vi "WILT Agilent Data To Main Display.vi"(0 "GUI Aisle 4":T3[](array[typedef]) {"Night Cycle Count" format="%04d"; "Day Cycle Count" format="%04d"}, 5 "GUI Aisle 3":T3[](array[typedef]) {"Night Cycle Count" format="%04d"; "Day Cycle Count" format="%04d"}, 7 "GUI Aisle 2":T3[](array[typedef]) {"Night Cycle Count" format="%04d"; "Day Cycle Count" format="%04d"}, 9 "GUI Aisle 1 (SLAT)":T3[](array[typedef]) {"Night Cycle Count" format="%04d"; "Day Cycle Count" format="%04d"}, 11 "Error In":errorcluster, 12 "GUI Aisle 1A (SLAT)":T3[](array[typedef]) {"Night Cycle Count" format="%04d"; "Day Cycle Count" format="%04d"}, 13 "Data Array":T1) -> (3 "Agilent Failure":bool, 4 "GUI Aisle 4 Out":T3[](array[typedef]) {"Night Cycle Count" format="%04d"; "Day Cycle Count" format="%04d"}, 6 "GUI Aisle 3 Out":T3[](array[typedef]) {"Night Cycle Count" format="%04d"; "Day Cycle Count" format="%04d"}, 8 "GUI Aisle 2 Out":T3[](array[typedef]) {"Night Cycle Count" format="%04d"; "Day Cycle Count" format="%04d"}, 10 "GUI Aisle 1 (SLAT) Out":T3[](array[typedef]) {"Night Cycle Count" format="%04d"; "Day Cycle Count" format="%04d"}, 14 "GUI Aisle 1A (SLAT) Out":T3[](array[typedef]) {"Night Cycle Count" format="%04d"; "Day Cycle Count" format="%04d"}, 15 "Error Out":errorcluster)   [LabVIEW 2016]
uses:
  Type Definitions/WILT Dryer.ctl
  Type Definitions/WILT Dryer Details.ctl
  Type Definitions/WILT Agilent Channel Definition.ctl
  Type Definitions/WILT DAQ Data.ctl
  Type Definitions/WILT Agilent Data Cluster.ctl
  Type Definitions/WILT Aisle Number.ctl
panel:
  in  "Test Data Only!!":T2[](array[typedef])=[{"Channel"="101", "Station"="1", "Label"="L1 Current", "Agilent Station"="1", "Data"=0.0}, {"Channel"="102", "Station"="1", "Label"="L2 Current", "Agilent Station"="1", "Data"=0.0}, {"Channel"="103", "Station"="2", "Label"="L1 Current", "Agilent Station"="1", "Data"=0.0}, {"Channel"="104", "Station"="2", "Label"="L2 Current", "Agilent Station"="1", "Data"=0.0}, {"Channel"="105", "Station"="3", "Label"="L1 Current", "Agilent Station"="1", "Data"=0.0}, {"Channel"="106", "Station"="3", "Label"="L2 Current", "Agilent Station"="1", "Data"=0.0}, {"Channel"="107", "Station"="4", "Label"="L1 Current", "Agilent Station"="1", "Data"=0.0}, {"Channel"="108", "Station"="4", "Label"="L2 Current", "Agilent Station"="1", "Data"=0.0}, {"Channel"="109", "Station"="5", "Label"="L1 Current", "Agilent Station"="1", "Data"=0.0}, {"Channel"="110", "Station"="5", "Label"="L2 Current", "Agilent Station"="1", "Data"=0.0}, {"Channel"="111", "Station"="6", "Label"="L1 Current", "Agilent Station"="1", "Data"=0.0}, {"Channel"="112", "Station"="6", "Label"="L2 Current", "Agilent Station"="1", "Data"=0.0}, {"Channel"="113", "Station"="7", "Label"="L1 Current", "Agilent Station"="1", "Data"=0.0}, {"Channel"="114", "Station"="7", "Label"="L2 Current", "Agilent Station"="1", "Data"=0.0}, {"Channel"="115", "Station"="8", "Label"="L1 Current", "Agilent Station"="1", "Data"=0.0}, {"Channel"="116", "Station"="8", "Label"="L2 Current", "Agilent Station"="1", "Data"=0.0}, {"Channel"="201", "Station"="9", "Label"="L1 Current", "Agilent Station"="1", "Data"=0.0}, {"Channel"="202", "Station"="9", "Label"="L2 Current", "Agilent Station"="1", "Data"=0.0}, {"Channel"="203", "Station"="10", "Label"="L1 Current", "Agilent Station"="1", "Data"=0.0}, {"Channel"="204", "Station"="10", "Label"="L2 Current", "Agilent Station"="1", "Data"=0.0}, {"Channel"="205", "Station"="11", "Label"="L1 Current", "Agilent Station"="1", "Data"=0.0}, {"Channel"="206", "Station"="11", "Label"="L2 Current", "Agilent Station"="1", "Data"=0.0}, {"Channel"="207", "Station"="12", "Label"="L1 Current", "Agilent Station"="1", "Data"=0.0}, {"Channel"="208", "Station"="12", "Label"="L2 Current", "Agilent Station"="1", "Data"=0.0}, {"Channel"="209", "Station"="13", "Label"="L1 Current", "Agilent Station"="1", "Data"=0.0}, {"Channel"="210", "Station"="13", "Label"="L2 Current", "Agilent Station"="1", "Data"=0.0}, {"Channel"="211", "Station"="14", "Label"="L1 Current", "Agilent Station"="1", "Data"=0.0}, {"Channel"="212", "Station"="14", "Label"="L2 Current", "Agilent Station"="1", "Data"=0.0}, {"Channel"="213", "Station"="15", "Label"="L1 Current", "Agilent Station"="1", "Data"=0.0}, {"Channel"="214", "Station"="15", "Label"="L2 Current", "Agilent Station"="1", "Data"=0.0}, {"Channel"="215", "Station"="16", "Label"="L1 Current", "Agilent Station"="1", "Data"=0.0}, {"Channel"="216", "Station"="16", "Label"="L2 Current", "Agilent Station"="1", "Data"=0.0}, {"Channel"="301", "Station"="17", "Label"="L1 Current", "Agilent Station"="1", "Data"=0.0}, {"Channel"="302", "Station"="17", "Label"="L2 Current", "Agilent Station"="1", "Data"=0.0}, {"Channel"="303", "Station"="18", "Label"="L1 Current", "Agilent Station"="1", "Data"=0.0}, {"Channel"="304", "Station"="18", "Label"="L2 Current", "Agilent Station"="1", "Data"=0.0}, {"Channel"="305", "Station"="19", "Label"="L1 Current", "Agilent Station"="1", "Data"=0.0}, {"Channel"="306", "Station"="19", "Label"="L2 Current", "Agilent Station"="1", "Data"=0.0}, {"Channel"="307", "Station"="20", "Label"="L1 Current", "Agilent Station"="1", "Data"=0.0}, {"Channel"="308", "Station"="20", "Label"="L2 Current", "Agilent Station"="1", "Data"=0.0}, {"Channel"="309", "Station"="21", "Label"="L1 Current", "Agilent Station"="1", "Data"=0.0}, {"Channel"="310", "Station"="21", "Label"="L2 Current", "Agilent Station"="1", "Data"=0.0}, {"Channel"="311", "Station"="22", "Label"="L1 Current", "Agilent Station"="1", "Data"=0.0}, {"Channel"="312", "Station"="22", "Label"="L2 Current", "Agilent Station"="1", "Data"=0.0}, {"Channel"="313", "Station"="23", "Label"="L1 Current", "Agilent Station"="1", "Data"=0.0}, {"Channel"="314", "Station"="23", "Label"="L2 Current", "Agilent Station"="1", "Data"=0.0}, {"Channel"="315", "Station"="24", "Label"="L1 Current", "Agilent Station"="1", "Data"=0.0}, {"Channel"="316", "Station"="24", "Label"="L2 Current", "Agilent Station"="1", "Data"=0.0}, {"Channel"="101", "Station"="25", "Label"="L1 Current", "Agilent Station"="2", "Data"=0.0}, {"Channel"="102", "Station"="25", "Label"="L2 Current", "Agilent Station"="2", "Data"=0.0}, {"Channel"="103", "Station"="26", "Label"="L1 Current", "Agilent Station"="2", "Data"=0.0}, {"Channel"="104", "Station"="26", "Label"="L2 Current", "Agilent Station"="2", "Data"=0.0}, {"Channel"="105", "Station"="27", "Label"="L1 Current", "Agilent Station"="2", "Data"=0.0}, {"Channel"="106", "Station"="27", "Label"="L2 Current", "Agilent Station"="2", "Data"=0.0}, {"Channel"="107", "Station"="28", "Label"="L1 Current", "Agilent Station"="2", "Data"=0.0}, {"Channel"="108", "Station"="28", "Label"="L2 Current", "Agilent Station"="2", "Data"=0.0}, {"Channel"="109", "Station"="29", "Label"="L1 Current", "Agilent Station"="2", "Data"=0.0}, {"Channel"="110", "Station"="29", "Label"="L2 Current", "Agilent Station"="2", "Data"=0.0}, {"Channel"="111", "Station"="30", "Label"="L1 Current", "Agilent Station"="2", "Data"=0.0}, {"Channel"="112", "Station"="30", "Label"="L2 Current", "Agilent Station"="2", "Data"=0.0}, {"Channel"="113", "Station"="31", "Label"="L1 Current", "Agilent Station"="2", "Data"=0.0}, {"Channel"="114", "Station"="31", "Label"="L2 Current", "Agilent Station"="2", "Data"=0.0}, {"Channel"="115", "Station"="32", "Label"="L1 Current", "Agilent Station"="2", "Data"=0.0}, {"Channel"="116", "Station"="32", "Label"="L2 Current", "Agilent Station"="2", "Data"=0.0}, {"Channel"="201", "Station"="5", "Label"="Volts", "Agilent Station"="2", "Data"=0.0}, {"Channel"="202", "Station"="6", "Label"="Volts", "Agilent Station"="2", "Data"=0.0}, {"Channel"="203", "Station"="7", "Label"="Volts", "Agilent Station"="2", "Data"=0.0}, {"Channel"="204", "Station"="8", "Label"="Volts", "Agilent Station"="2", "Data"=0.0}, {"Channel"="205", "Station"="9", "Label"="Volts", "Agilent Station"="2", "Data"=0.0}, {"Channel"="206", "Station"="10", "Label"="Volts", "Agilent Station"="2", "Data"=0.0}, {"Channel"="207", "Station"="11", "Label"="Volts", "Agilent Station"="2", "Data"=0.0}, {"Channel"="208", "Station"="12", "Label"="Volts", "Agilent Station"="2", "Data"=0.0}, {"Channel"="209", "Station"="13", "Label"="Volts", "Agilent Station"="2", "Data"=0.0}, {"Channel"="210", "Station"="14", "Label"="Volts", "Agilent Station"="2", "Data"=0.0}, {"Channel"="211", "Station"="21-23", "Label"="Volts", "Agilent Station"="2", "Data"=0.0}, {"Channel"="212", "Station"="24-26", "Label"="Volts", "Agilent Station"="2", "Data"=0.0}, {"Channel"="213", "Station"="27-29", "Label"="Volts", "Agilent Station"="2", "Data"=0.0}, {"Channel"="214", "Station"="30-32", "Label"="Volts", "Agilent Station"="2", "Data"=0.0}, {"Channel"="215", "Station"="15", "Label"="Volts", "Agilent Station"="2", "Data"=0.0}, {"Channel"="216", "Station"="16", "Label"="Volts", "Agilent Station"="2", "Data"=0.0}, {"Channel"="201", "Station"="1", "Label"="Temperature", "Agilent Station"="3", "Data"=0.0}, {"Channel"="202", "Station"="2", "Label"="Temperature", "Agilent Station"="3", "Data"=0.0}, {"Channel"="203", "Station"="3", "Label"="Temperature", "Agilent Station"="3", "Data"=0.0}, {"Channel"="204", "Station"="4", "Label"="Temperature", "Agilent Station"="3", "Data"=0.0}, {"Channel"="205", "Station"="5", "Label"="Temperature", "Agilent Station"="3", "Data"=0.0}, {"Channel"="206", "Station"="6", "Label"="Temperature", "Agilent Station"="3", "Data"=0.0}, {"Channel"="207", "Station"="7", "Label"="Temperature", "Agilent Station"="3", "Data"=0.0}, {"Channel"="208", "Station"="8", "Label"="Temperature", "Agilent Station"="3", "Data"=0.0}, {"Channel"="209", "Station"="9", "Label"="Temperature", "Agilent Station"="3", "Data"=0.0}, {"Channel"="210", "Station"="10", "Label"="Temperature", "Agilent Station"="3", "Data"=0.0}, {"Channel"="211", "Station"="11", "Label"="Temperature", "Agilent Station"="3", "Data"=0.0}, {"Channel"="212", "Station"="12", "Label"="Temperature", "Agilent Station"="3", "Data"=0.0}, {"Channel"="213", "Station"="13", "Label"="Temperature", "Agilent Station"="3", "Data"=0.0}, {"Channel"="214", "Station"="14", "Label"="Temperature", "Agilent Station"="3", "Data"=0.0}, {"Channel"="215", "Station"="15", "Label"="Temperature", "Agilent Station"="3", "Data"=0.0}, {"Channel"="216", "Station"="16", "Label"="Temperature", "Agilent Station"="3", "Data"=0.0}, {"Channel"="217", "Station"="17", "Label"="Temperature", "Agilent Station"="3", "Data"=0.0}, {"Channel"="218", "Station"="18", "Label"="Temperature", "Agilent Station"="3", "Data"=0.0}, {"Channel"="219", "Station"="19", "Label"="Temperature", "Agilent Station"="3", "Data"=0.0}, {"Channel"="220", "Station"="20", "Label"="Temperature", "Agilent Station"="3", "Data"=0.0}, {"Channel"="301", "Station"="21", "Label"="Temperature", "Agilent Station"="3", "Data"=0.0}, {"Channel"="302", "Station"="22", "Label"="Temperature", "Agilent Station"="3", "Data"=0.0}, {"Channel"="303", "Station"="23", "Label"="Temperature", "Agilent Station"="3", "Data"=0.0}, {"Channel"="304", "Station"="24", "Label"="Temperature", "Agilent Station"="3", "Data"=0.0}, {"Channel"="305", "Station"="25", "Label"="Temperature", "Agilent Station"="3", "Data"=0.0}, {"Channel"="306", "Station"="26", "Label"="Temperature", "Agilent Station"="3", "Data"=0.0}, {"Channel"="307", "Station"="27", "Label"="Temperature", "Agilent Station"="3", "Data"=0.0}, {"Channel"="308", "Station"="28", "Label"="Temperature", "Agilent Station"="3", "Data"=0.0}, {"Channel"="309", "Station"="29", "Label"="Temperature", "Agilent Station"="3", "Data"=0.0}, {"Channel"="310", "Station"="30", "Label"="Temperature", "Agilent Station"="3", "Data"=0.0}, {"Channel"="311", "Station"="31", "Label"="Temperature", "Agilent Station"="3", "Data"=0.0}, {"Channel"="312", "Station"="32", "Label"="Temperature", "Agilent Station"="3", "Data"=0.0}, {"Channel"="313", "Station"="1", "Label"="Volts", "Agilent Station"="3", "Data"=0.0}, {"Channel"="314", "Station"="2", "Label"="Volts", "Agilent Station"="3", "Data"=0.0}, {"Channel"="315", "Station"="3", "Label"="Volts", "Agilent Station"="3", "Data"=0.0}, {"Channel"="316", "Station"="4", "Label"="Volts", "Agilent Station"="3", "Data"=0.0}, {"Channel"="101", "Station"="33", "Label"="L1 Current", "Agilent Station"="4", "Data"=0.0}, {"Channel"="102", "Station"="33", "Label"="L2 Current", "Agilent Station"="4", "Data"=0.0}, {"Channel"="103", "Station"="34", "Label"="L1 Current", "Agilent Station"="4", "Data"=0.0}, {"Channel"="104", "Station"="34", "Label"="L2 Current", "Agilent Station"="4", "Data"=0.0}, {"Channel"="105", "Station"="35", "Label"="L1 Current", "Agilent Station"="4", "Data"=0.0}, {"Channel"="106", "Station"="35", "Label"="L2 Current", "Agilent Station"="4", "Data"=0.0}, {"Channel"="107", "Station"="36", "Label"="L1 Current", "Agilent Station"="4", "Data"=0.0}, {"Channel"="108", "Station"="36", "Label"="L2 Current", "Agilent Station"="4", "Data"=0.0}, {"Channel"="109", "Station"="37", "Label"="L1 Current", "Agilent Station"="4", "Data"=0.0}, {"Channel"="110", "Station"="37", "Label"="L2 Current", "Agilent Station"="4", "Data"=0.0}, {"Channel"="111", "Station"="38", "Label"="L1 Current", "Agilent Station"="4", "Data"=0.0}, {"Channel"="112", "Station"="38", "Label"="L2 Current", "Agilent Station"="4", "Data"=0.0}, {"Channel"="113", "Station"="39", "Label"="L1 Current", "Agilent Station"="4", "Data"=0.0}, {"Channel"="114", "Station"="39", "Label"="L2 Current", "Agilent Station"="4", "Data"=0.0}, {"Channel"="115", "Station"="40", "Label"="L1 Current", "Agilent Station"="4", "Data"=0.0}, {"Channel"="116", "Station"="40", "Label"="L2 Current", "Agilent Station"="4", "Data"=0.0}, {"Channel"="201", "Station"="41", "Label"="L1 Current", "Agilent Station"="4", "Data"=0.0}, {"Channel"="202", "Station"="41", "Label"="L2 Current", "Agilent Station"="4", "Data"=0.0}, {"Channel"="203", "Station"="42", "Label"="L1 Current", "Agilent Station"="4", "Data"=0.0}, {"Channel"="204", "Station"="42", "Label"="L2 Current", "Agilent Station"="4", "Data"=0.0}, {"Channel"="205", "Station"="43", "Label"="L1 Current", "Agilent Station"="4", "Data"=0.0}, {"Channel"="206", "Station"="43", "Label"="L2 Current", "Agilent Station"="4", "Data"=0.0}, {"Channel"="207", "Station"="44", "Label"="L1 Current", "Agilent Station"="4", "Data"=0.0}, {"Channel"="208", "Station"="44", "Label"="L2 Current", "Agilent Station"="4", "Data"=0.0}, {"Channel"="209", "Station"="45", "Label"="L1 Current", "Agilent Station"="4", "Data"=0.0}, {"Channel"="210", "Station"="45", "Label"="L2 Current", "Agilent Station"="4", "Data"=0.0}, {"Channel"="211", "Station"="46", "Label"="L1 Current", "Agilent Station"="4", "Data"=0.0}, {"Channel"="212", "Station"="46", "Label"="L2 Current", "Agilent Station"="4", "Data"=0.0}, {"Channel"="213", "Station"="47", "Label"="L1 Current", "Agilent Station"="4", "Data"=0.0}, {"Channel"="214", "Station"="47", "Label"="L2 Current", "Agilent Station"="4", "Data"=0.0}, {"Channel"="215", "Station"="48", "Label"="L1 Current", "Agilent Station"="4", "Data"=0.0}, {"Channel"="216", "Station"="48", "Label"="L2 Current", "Agilent Station"="4", "Data"=0.0}, {"Channel"="301", "Station"="49", "Label"="L1 Current", "Agilent Station"="4", "Data"=0.0}, {"Channel"="302", "Station"="49", "Label"="L2 Current", "Agilent Station"="4", "Data"=0.0}, {"Channel"="303", "Station"="50", "Label"="L1 Current", "Agilent Station"="4", "Data"=0.0}, {"Channel"="304", "Station"="50", "Label"="L2 Current", "Agilent Station"="4", "Data"=0.0}, {"Channel"="305", "Station"="51", "Label"="L1 Current", "Agilent Station"="4", "Data"=0.0}, {"Channel"="306", "Station"="51", "Label"="L2 Current", "Agilent Station"="4", "Data"=0.0}, {"Channel"="307", "Station"="52", "Label"="L1 Current", "Agilent Station"="4", "Data"=0.0}, {"Channel"="308", "Station"="52", "Label"="L2 Current", "Agilent Station"="4", "Data"=0.0}, {"Channel"="309", "Station"="53", "Label"="L1 Current", "Agilent Station"="4", "Data"=0.0}, {"Channel"="310", "Station"="53", "Label"="L2 Current", "Agilent Station"="4", "Data"=0.0}, {"Channel"="311", "Station"="54", "Label"="L1 Current", "Agilent Station"="4", "Data"=0.0}, {"Channel"="312", "Station"="54", "Label"="L2 Current", "Agilent Station"="4", "Data"=0.0}, {"Channel"="313", "Station"="55", "Label"="L1 Current", "Agilent Station"="4", "Data"=0.0}, {"Channel"="314", "Station"="55", "Label"="L2 Current", "Agilent Station"="4", "Data"=0.0}, {"Channel"="315", "Station"="56", "Label"="L1 Current", "Agilent Station"="4", "Data"=0.0}, {"Channel"="316", "Station"="56", "Label"="L2 Current", "Agilent Station"="4", "Data"=0.0}, {"Channel"="101", "Station"="33", "Label"="Temperature", "Agilent Station"="6", "Data"=0.0}, {"Channel"="102", "Station"="34", "Label"="Temperature", "Agilent Station"="6", "Data"=0.0}, {"Channel"="103", "Station"="35", "Label"="Temperature", "Agilent Station"="6", "Data"=0.0}, {"Channel"="104", "Station"="36", "Label"="Temperature", "Agilent Station"="6", "Data"=0.0}, {"Channel"="105", "Station"="37", "Label"="Temperature", "Agilent Station"="6", "Data"=0.0}, {"Channel"="106", "Station"="38", "Label"="Temperature", "Agilent Station"="6", "Data"=0.0}, {"Channel"="107", "Station"="39", "Label"="Temperature", "Agilent Station"="6", "Data"=0.0}, {"Channel"="108", "Station"="40", "Label"="Temperature", "Agilent Station"="6", "Data"=0.0}, {"Channel"="109", "Station"="41", "Label"="Temperature", "Agilent Station"="6", "Data"=0.0}, {"Channel"="110", "Station"="42", "Label"="Temperature", "Agilent Station"="6", "Data"=0.0}, {"Channel"="111", "Station"="43", "Label"="Temperature", "Agilent Station"="6", "Data"=0.0}, {"Channel"="112", "Station"="44", "Label"="Temperature", "Agilent Station"="6", "Data"=0.0}, {"Channel"="113", "Station"="45", "Label"="Temperature", "Agilent Station"="6", "Data"=0.0}, {"Channel"="114", "Station"="46", "Label"="Temperature", "Agilent Station"="6", "Data"=0.0}, {"Channel"="115", "Station"="47", "Label"="Temperature", "Agilent Station"="6", "Data"=0.0}, {"Channel"="116", "Station"="48", "Label"="Temperature", "Agilent Station"="6", "Data"=0.0}, {"Channel"="117", "Station"="49", "Label"="Temperature", "Agilent Station"="6", "Data"=0.0}, {"Channel"="118", "Station"="50", "Label"="Temperature", "Agilent Station"="6", "Data"=0.0}, {"Channel"="119", "Station"="51", "Label"="Temperature", "Agilent Station"="6", "Data"=0.0}, {"Channel"="120", "Station"="52", "Label"="Temperature", "Agilent Station"="6", "Data"=0.0}, {"Channel"="201", "Station"="53", "Label"="Temperature", "Agilent Station"="6", "Data"=0.0}, {"Channel"="202", "Station"="54", "Label"="Temperature", "Agilent Station"="6", "Data"=0.0}, {"Channel"="203", "Station"="55", "Label"="Temperature", "Agilent Station"="6", "Data"=0.0}, {"Channel"="204", "Station"="56", "Label"="Temperature", "Agilent Station"="6", "Data"=0.0}, {"Channel"="205", "Station"="33-35", "Label"="Volts", "Agilent Station"="6", "Data"=0.0}, {"Channel"="206", "Station"="36-38", "Label"="Volts", "Agilent Station"="6", "Data"=0.0}, {"Channel"="207", "Station"="39-40", "Label"="Volts", "Agilent Station"="6", "Data"=0.0}, {"Channel"="208", "Station"="42-44", "Label"="Volts", "Agilent Station"="6", "Data"=0.0}, {"Channel"="209", "Station"="45-47", "Label"="Volts", "Agilent Station"="6", "Data"=0.0}, {"Channel"="210", "Station"="45", "Label"="Volts (208)", "Agilent Station"="6", "Data"=0.0}, {"Channel"="211", "Station"="45", "Label"="SW (208)", "Agilent Station"="6", "Data"=0.0}, {"Channel"="212", "Station"="48-50", "Label"="Volts", "Agilent Station"="6", "Data"=0.0}, {"Channel"="213", "Station"="48", "Label"="SW (208)", "Agilent Station"="6", "Data"=0.0}, {"Channel"="214", "Station"="51", "Label"="Volts (208)", "Agilent Station"="6", "Data"=0.0}, {"Channel"="215", "Station"="51", "Label"="SW (208)", "Agilent Station"="6", "Data"=0.0}, {"Channel"="216", "Station"="54-56", "Label"="Volts", "Agilent Station"="6", "Data"=0.0}, {"Channel"="301", "Station"="17", "Label"="Volts", "Agilent Station"="6", "Data"=0.0}, {"Channel"="302", "Station"="18", "Label"="Volts", "Agilent Station"="6", "Data"=0.0}, {"Channel"="303", "Station"="19", "Label"="Volts", "Agilent Station"="6", "Data"=0.0}, {"Channel"="304", "Station"="20", "Label"="Volts", "Agilent Station"="6", "Data"=0.0}, {"Channel"="305", "Station"="51-53", "Label"="Volts", "Agilent Station"="6", "Data"=0.0}, {"Channel"="306", "Station"="48", "Label"="Volts (208)", "Agilent Station"="6", "Data"=0.0}]
  # "Day"
  # "Night"
  # "Day"
  # "Night"
  # "Day"
  # "Night"
  # "Day"
  # "Night"
  # "Day"
  # "Night"
  # "Day"
  # "Night"
  # "Day"
  # "Night"
  # "Day"
  # "Night"
  # "Day"
  # "Night"
  # "Day"
  # "Night"
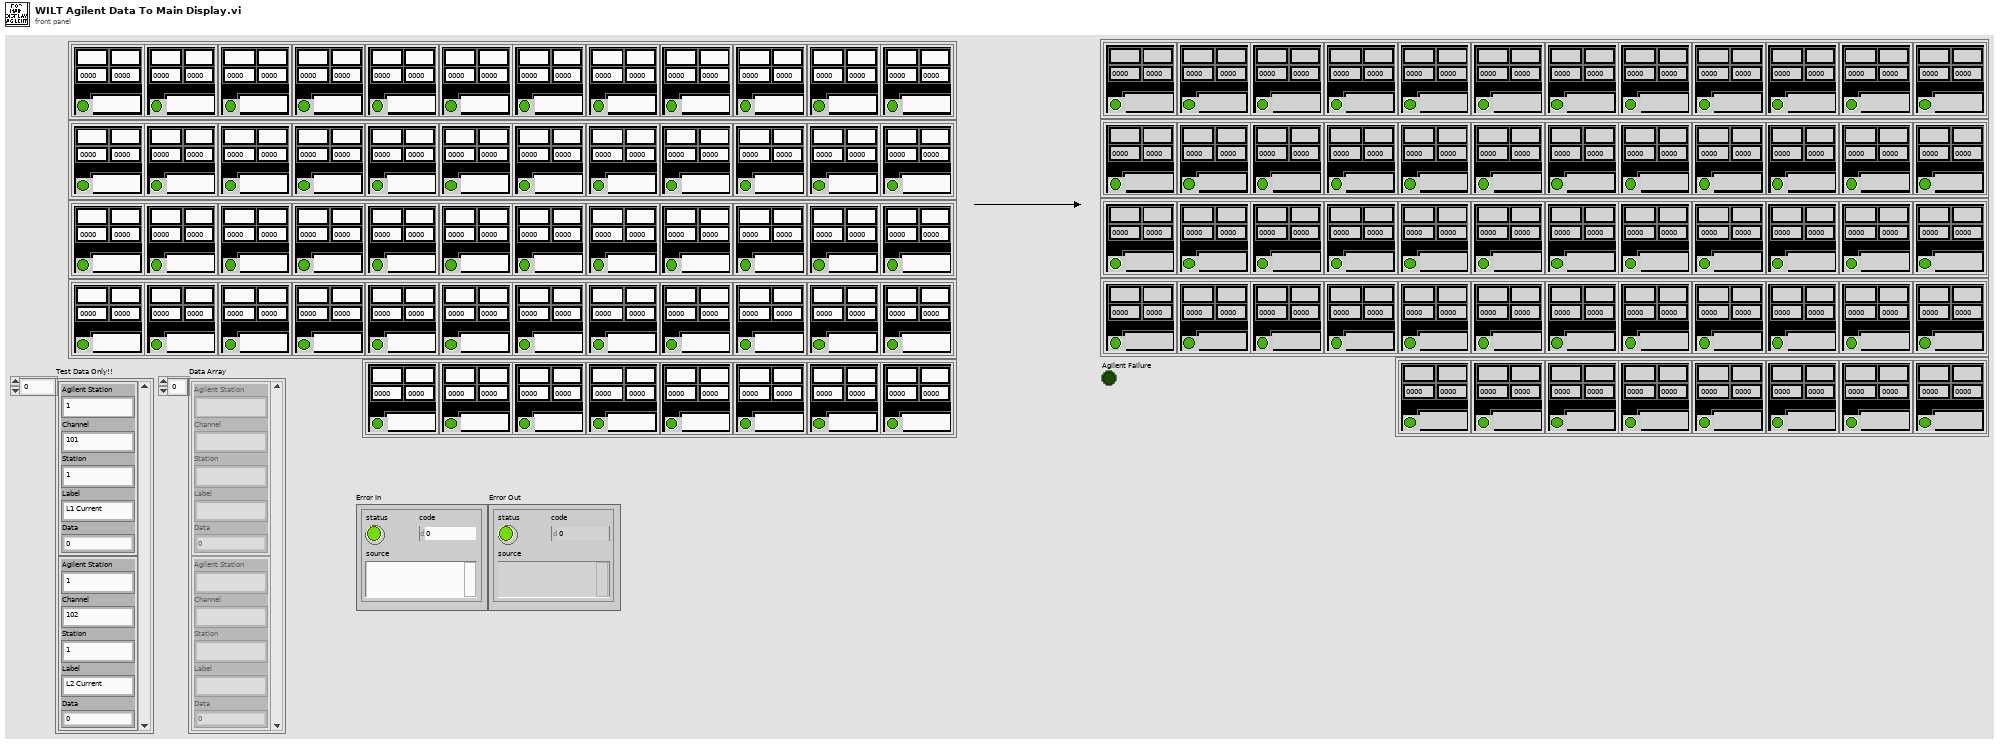
[diagram p1: front panel]
types:
  T1 = typedef "WILT Agilent Data Cluster.ctl" = T2[]
  T2 = typedef "WILT Agilent Channel Definition.ctl" = cluster{"Channel":string, "Station":string, "Label":string, "Agilent Station":string, "Data":dbl}
  T3 = typedef "WILT Dryer.ctl" = cluster{"Lab ID":string, "Day Cycle Count":i32, "Station Label":string, "Dryer Details":T4, "Status Color":u32, "Invisible Button":bool, "Night Cycle Count":i32, "Station Index":i32, "Cycle Index":string, "Audit Alert":bool, "Agilent Channel Definition":T2, "DAQ Data":T5}
  T4 = typedef "WILT Dryer Details.ctl" = cluster{"Station":string, "Lab ID":string, "TR Number":string}
  T5 = typedef "WILT DAQ Data.ctl" = cluster{"L1 Current":dbl, "L2 Current":dbl, "Temperature  Deg F (TC)":dbl, "Volts":dbl, "Volts (208)":dbl, "SW (208)":dbl}
  T6 = typedef "WILT Aisle Number.ctl" = enum16{"Aisle 4", "Aisle 3", "Aisle 2", "Aisle 1A", "Aisle 1"}
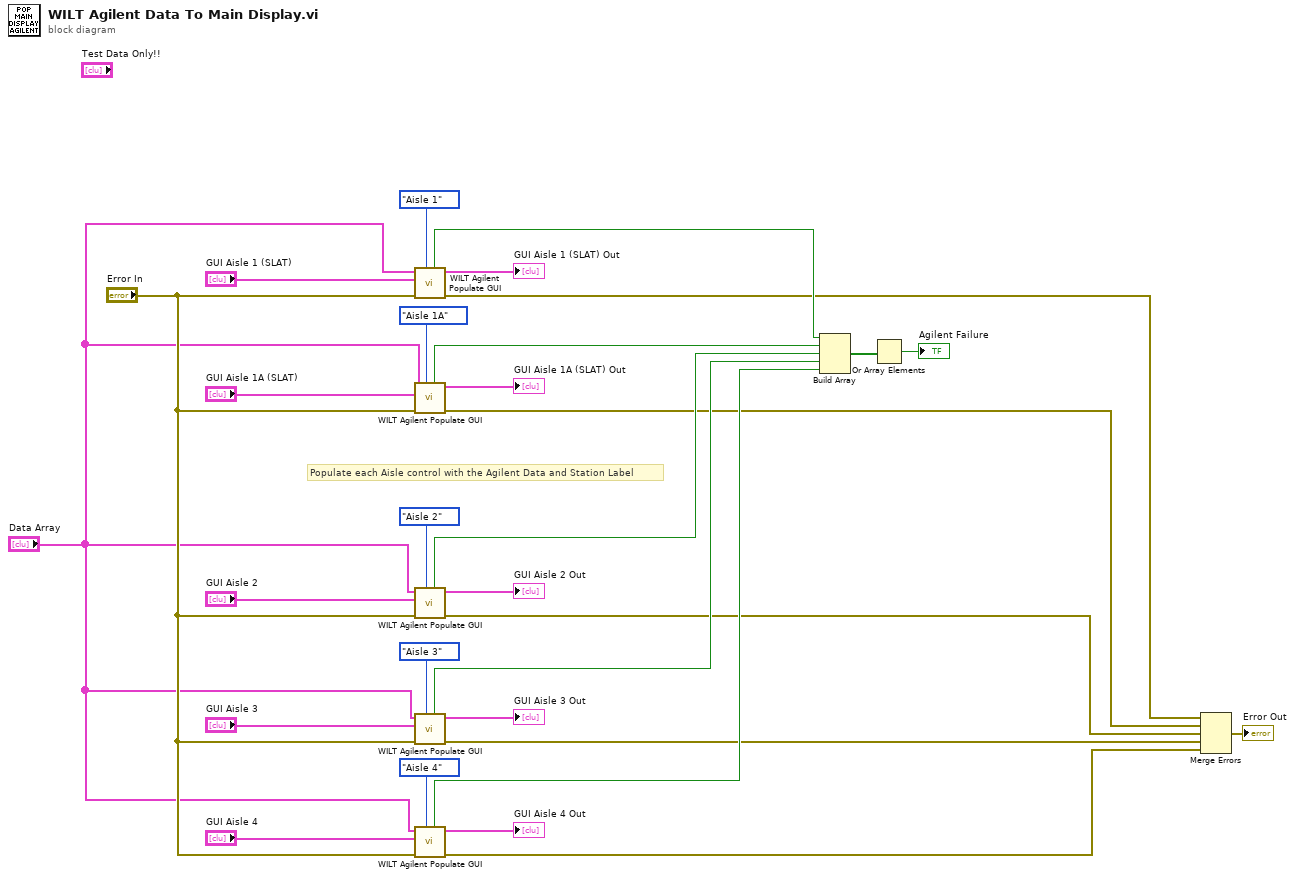
[diagram p0: block diagram]
diagram:
  # "Populate each Aisle control with the Agilent Data and Station Label"
  n1 = call "WILT Agilent Populate GUI.vi"("Aisle Number"=WILT_Aisle_Number."Aisle 1", "Error In"="Error In", "GUI Aisle Input"="GUI Aisle 1 (SLAT)", "Data Array"="Data Array") -> ("Error Out"=w5:errorcluster, "GUI Aisle Output"=→"GUI Aisle 1 (SLAT) Out":T3[], "Agilent Failure"=w12:bool)  [unwired: 5 in]
  n2 = call "WILT Agilent Populate GUI.vi"("Aisle Number"=WILT_Aisle_Number."Aisle 1A", "Error In"="Error In", "GUI Aisle Input"="GUI Aisle 1A (SLAT)", "Data Array"="Data Array") -> ("Error Out"=w4:errorcluster, "GUI Aisle Output"=→"GUI Aisle 1A (SLAT) Out":T3[], "Agilent Failure"=w11:bool)  [unwired: 5 in]
  n3 = call "WILT Agilent Populate GUI.vi"("Aisle Number"=WILT_Aisle_Number."Aisle 2", "Error In"="Error In", "GUI Aisle Input"="GUI Aisle 2", "Data Array"="Data Array") -> ("Error Out"=w3:errorcluster, "GUI Aisle Output"=→"GUI Aisle 2 Out":T3[], "Agilent Failure"=w8:bool)  [unwired: 5 in]
  n4 = call "WILT Agilent Populate GUI.vi"("Aisle Number"=WILT_Aisle_Number."Aisle 3", "Error In"="Error In", "GUI Aisle Input"="GUI Aisle 3", "Data Array"="Data Array") -> ("Error Out"=w2:errorcluster, "GUI Aisle Output"=→"GUI Aisle 3 Out":T3[], "Agilent Failure"=w7:bool)  [unwired: 5 in]
  n5 = call "WILT Agilent Populate GUI.vi"("Aisle Number"=WILT_Aisle_Number."Aisle 4", "Error In"="Error In", "GUI Aisle Input"="GUI Aisle 4", "Data Array"="Data Array") -> ("Error Out"=w1:errorcluster, "GUI Aisle Output"=→"GUI Aisle 4 Out":T3[], "Agilent Failure"=w6:bool)  [unwired: 5 in]
  n6 = Build Array(w12, w11, w8, w7, w6) -> (w10:bool[])
  n7 = Or Array Elements(Boolean array=w10) -> (logical OR=→"Agilent Failure":bool)
  n8 = Merge Errors(w5, w4, w3, w2, w1) -> (→"Error Out":errorcluster)
